vi "GetChildByIndex.vi"(8 "error in (no error)":errorcluster, 10 "Index(0)":i32, 11 "BrowerComponent in":refnum<class "BrowerComponent.lvclass">) -> (0 "error out":errorcluster, 2 "BrowerComponent":refnum<class "BrowerComponent.lvclass">, 3 "BrowerComponent out":refnum<class "BrowerComponent.lvclass">)   [LabVIEW 2015, in "BrowerComponent.lvclass"]
uses:
  BrowerComponent.lvclass
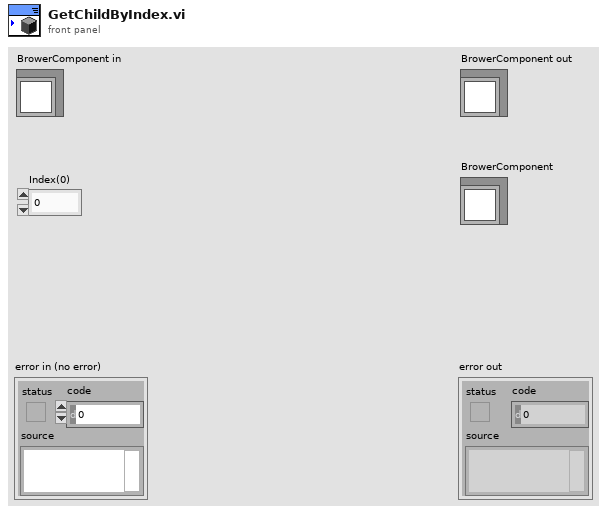
[diagram p1: front panel]
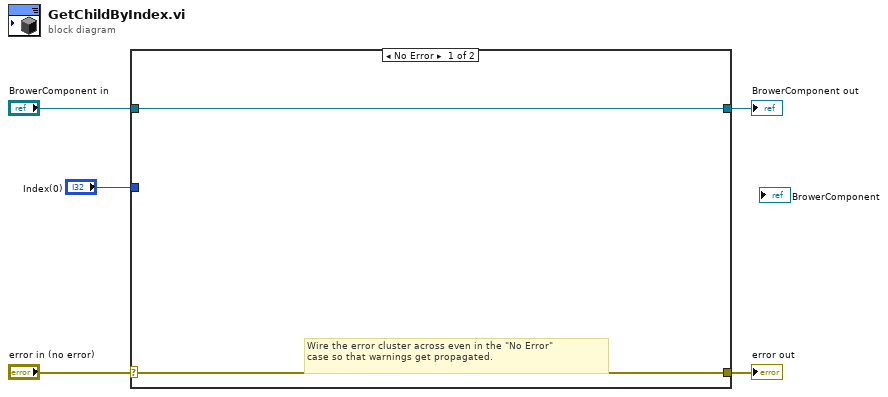
[diagram p0: block diagram]
diagram:
  n1 = case shown="No Error" "error in (no error)" {
    selector: "error in (no error)" -> [w6 w9]
    tunnel: [w6 w9] -> w4
    tunnel: [w7 w8] -> w2
    tunnel: "BrowerComponent in" -> [w7 w8]
    tunnel: "Index(0)" -> [_ _]
    frame No Error {
      # "Wire the error cluster across even in the \"No Error\"\ncase so that warnings get propagated."
    }
    frame Error {
    }
  }
  "error out" <- w4
  "BrowerComponent out" <- w2
